vi "Test.vi"() -> ()   [LabVIEW 2019]
panel:
  out "childs":string[](array[string])
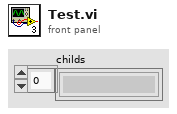
[diagram p1: front panel]
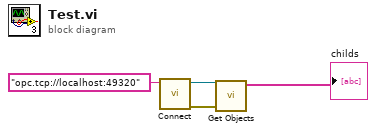
[diagram p0: block diagram]
diagram:
  n1 = call "Connect.vi"("OPC UA ENDpoint"="opc.tcp://localhost:49320") -> ("error out"=w4:errorcluster, "session out"=w3:refnum<k35>)  [unwired: 7 in, 2 out]
  n2 = call "Get Objects.vi"("error in (no error)"=w4, "session in"=w3) -> ("childs"=→"childs":string[])  [unwired: 8 in, 1 out]
